vi "CalcArea.vi"(11 "Cluster":T1) -> (3 "Numeric":u64)   [LabVIEW 2023, in "2024_12.lvclass"]
uses:
  2024_12.lvclass
  2024_12.lvclass/2024_12.ctl
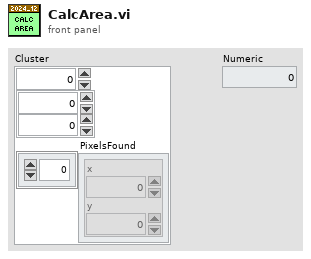
[diagram p1: front panel]
types:
  T1 = cluster{"Numeric":u8, "Cluster":cluster{"Numeric":i32, "Numeric":i32}, "PixelsFound":cluster{"x":i32, "y":i32}[]}
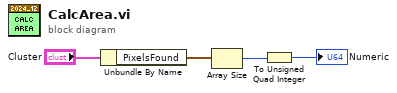
[diagram p0: block diagram]
diagram:
  n1 = Unbundle By Name("Cluster") -> ("PixelsFound"=w3:cluster{"x":i32, "y":i32}[])
  n2 = Array Size(array=w3) -> (size(s)=w2:i32)
  n3 = To Unsigned Quad Integer(1:w2) -> (0:→"Numeric":u64)
